vi "spectrum_fundamental.vi"() -> ()   [LabVIEW 2023]
uses:
  <vilib>/measure/matone.llb/Extract Single Tone Information N Chan.vi
  <vilib>/express/express analysis/Spectral/XNode/ExpressSpectralMeasurementsBlockNode.xnode
  <vilib>/measure/NI_MAPro.lvlib
  <vilib>/express/express analysis/Spectral/Block/exnSpectralBlock spectral measurements RMS poly.vi
  <vilib>/express/express analysis/Spectral/Block/exnSpectralBlock spectral measurements RMS DDT.vi
panel:
  in  "Frequency (Hz)":dbl=10.1 caption="Frequency"
  in  "Entered Freq":bool
  in  "Duration (s)":dbl=1.0
  out "Raw Waveform":dynamicdata(graph)
  out "Past Frequencies":i32[](array[numeric])
  out "Last Freq (Hz)":i32
  in  "Play":bool
  in  "stop":bool
  in  "Record":bool
  out "Power Spectrum":dynamicdata(graph)
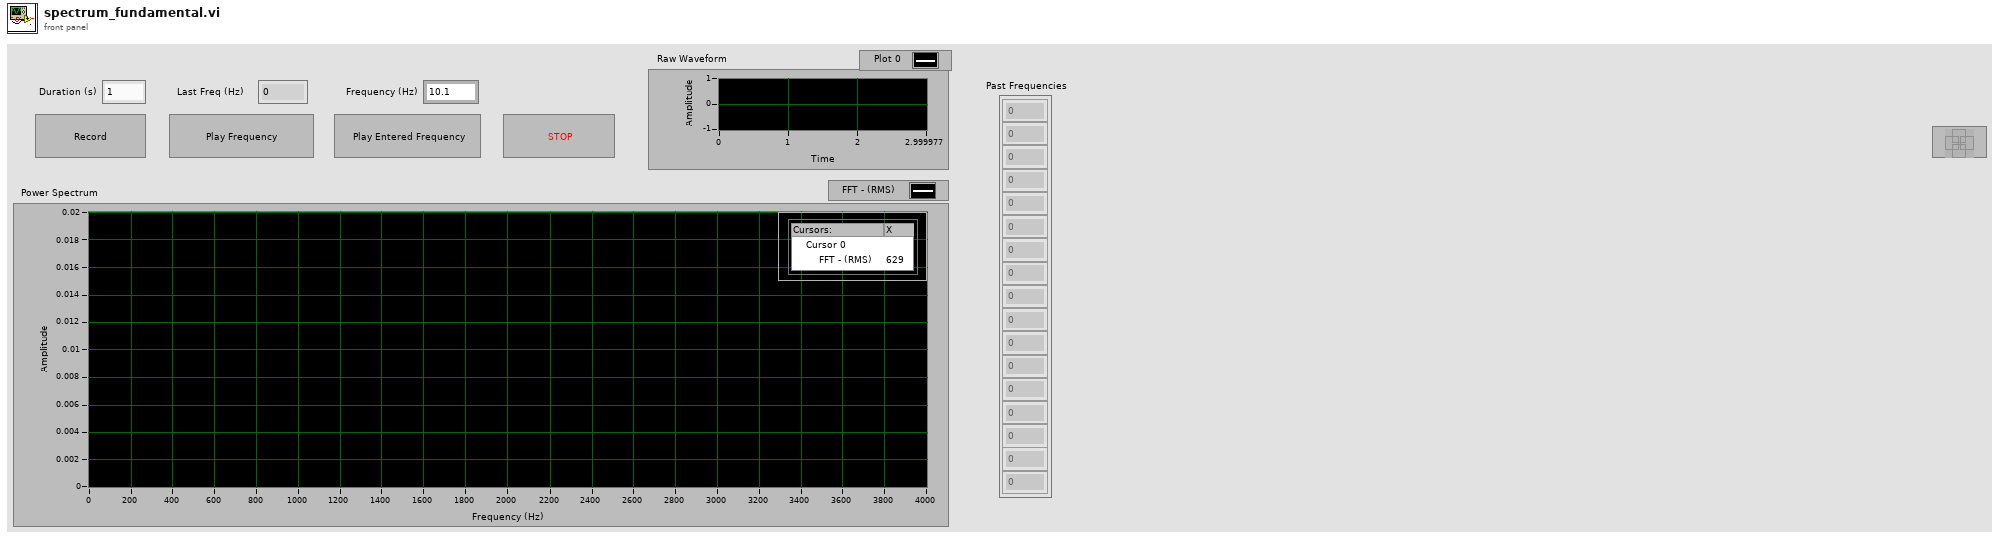
[diagram p1: front panel]
types:
  T1 = cluster{"averaging mode":u16, "weighting mode":u16, "number of averages":u32}
  T2 = cluster{"dB On (F)":bool, "unwrap phase (F)":bool, "convert to degree (F)":bool}
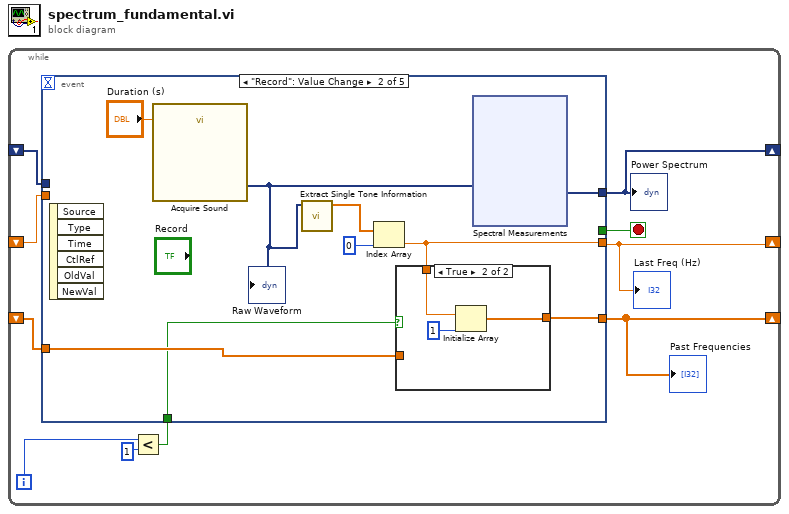
[diagram p0: block diagram]
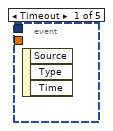
[diagram p2: hidden frame]
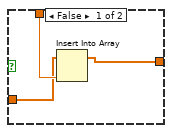
[diagram p3: hidden frame]
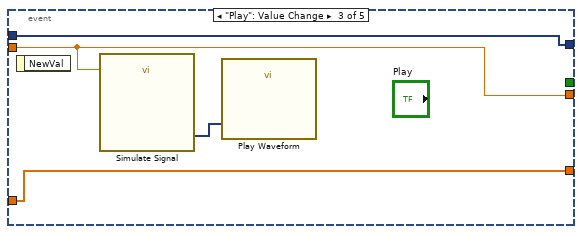
[diagram p4: hidden frame]
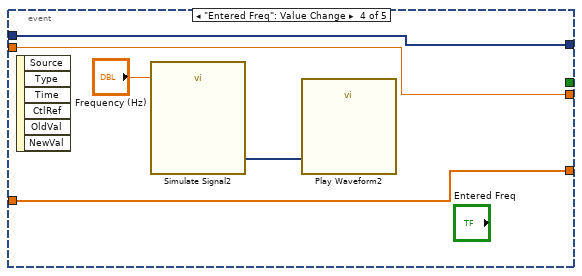
[diagram p5: hidden frame]
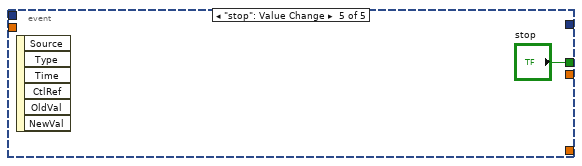
[diagram p6: hidden frame]
diagram:
  n1 = while {
    shift-right: [w8] -> _
    shift-left: _ -> [w10]
    shift-right: [w2] -> _
    shift-left: _ -> [w7]
    shift-right: [w1] -> _
    shift-left: _ -> [w4]
    i -> [w6]
    stop <- w9 stop-if-true
    n2 = Less?(x=w6, y=1) -> (x < y?=w3:bool)
    n3 = event shown="[1] \"Record\": Value Change" {
      selector: _ -> [_ _ _ _ _]
      dyn-events: _ -> [_ _ _ _ _]
      timeout: _ -> [_ _ _ _ _]
      tunnel: [_ w19 w39 w41 _] -> w8
      tunnel: w10 -> [_ _ w39 w41 _]
      tunnel: [_ _ _ _ "stop"] -> w9
      tunnel: w7 -> [_ _ w36 w42 _]
      tunnel: [_ w12 w36 w42 _] -> w2
      tunnel: [_ w16 w37 w43 _] -> w1
      tunnel: w4 -> [_ w18 w37 w43 _]
      tunnel: w3 -> [_ w17 _ _ _]
      event Timeout {
        n4 = event-data() -> ()  [unwired: 1 in, 3 out]
      }
      event "Record": Value Change {
        n5 = event-data() -> ()  [unwired: 1 in, 6 out]
        n6 = call "Acquire Sound"("Duration (s)"="Duration (s)") -> ("Data"=w14:dynamicdata)  [unwired: 17 in, 1 out]
        "Raw Waveform" <- w14
        n7 = call-poly <vilib>:"Extract Single Tone Information.vi"("time signals in"=w14) -> ("detected frequencies"=w13:dbl[])  [unwired: 5 in, 5 out]
        n8 = Index Array(array=w13, index=0) -> (element=w12:dbl)
        n9 = case shown="True" w17 {
          tunnel: [w22 w23] -> w16
          tunnel: w18 -> [w20 _]
          tunnel: w12 -> [w21 w25]
          frame False {
            n10 = Insert Into Array(array=w20, new element=w21) -> (w22:dbl[])  [unwired: 1 in]
          }
          frame True {
            n11 = Initialize Array(w25, 1) -> (w23:dbl[])
          }
        }
        n12 = xnode "Spectral Measurements"("Signals"=w14) -> ("FFT - (RMS)"=w19:dynamicdata)  [unwired: 1 in, 2 out]
      }
      event "Play": Value Change {
        n13 = event-data() -> ()  [unwired: 1 in, 1 out]
        n14 = call "Simulate Signal"("Frequency"=w36) -> ("Sine"=w38:dynamicdata)  [unwired: 13 in, 1 out]
        n15 = call "Play Waveform"("Data"=w38) -> ()  [unwired: 18 in, 1 out]
      }
      event "Entered Freq": Value Change {
        n16 = event-data() -> ()  [unwired: 1 in, 6 out]
        n17 = call "Simulate Signal2"("Frequency"="Frequency (Hz)") -> ("Sine"=w44:dynamicdata)  [unwired: 13 in, 1 out]
        n18 = call "Play Waveform2"("Data"=w44) -> ()  [unwired: 18 in, 1 out]
      }
      event "stop": Value Change {
        n19 = event-data() -> ()  [unwired: 1 in, 6 out]
      }
    }
    "Power Spectrum" <- w8
    "Last Freq (Hz)" <- w2
    "Past Frequencies" <- w1
  }
